vi "Release.vi"(8 "error in (no error)":errorcluster, 11 "Instance":T1) -> (0 "error out":errorcluster, 3 "Children":i32[](array[numeric]))   [LabVIEW 2022 SP3, in "Shared.lvlib"]
uses:
  Shared.lvlib
  Controls/Instance.ctl
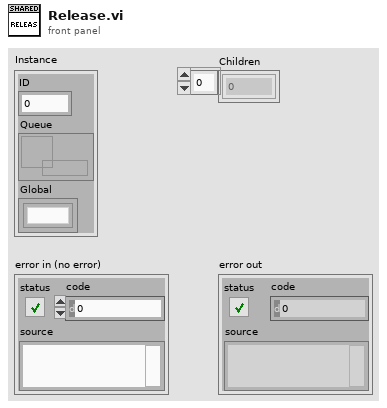
[diagram p1: front panel]
types:
  T1 = typedef "Shared.lvlib/Instance.ctl" = cluster{"ID":i32, "Queue":refnum<queue>, "Global":refnum<k1>}
  T2 = cluster{"ID":i32, "Name":string, "Parent":i32, "Queue":refnum<queue>, "Ini Path":path, "Ini Section":string, "VI Name":string, "VI Path":path, "VI Refnum":refnum<vi>, "Group":string}[]
  T3 = cluster{"ID":i32, "Name":string, "Parent":i32, "Queue":refnum<queue>, "Ini Path":path, "Ini Section":string, "VI Name":string, "VI Path":path, "VI Refnum":refnum<vi>, "Group":string}
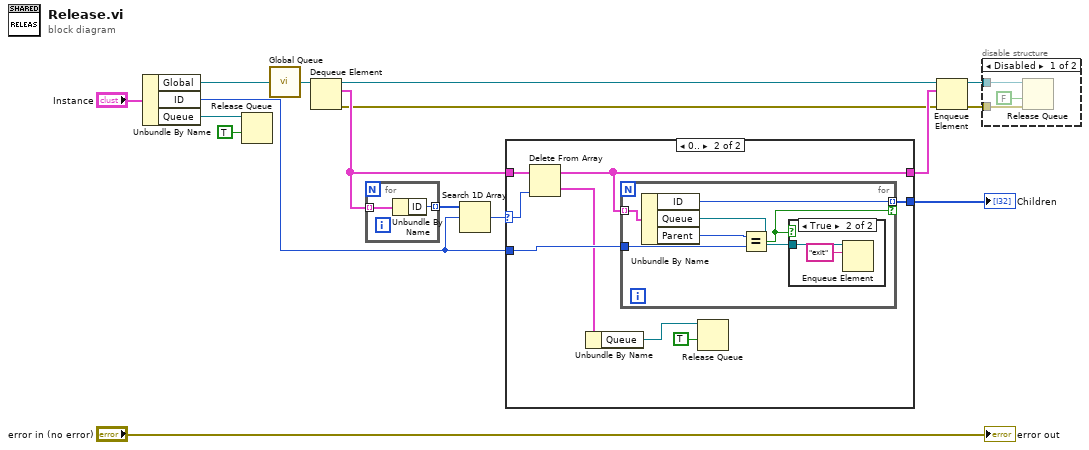
[diagram p0: block diagram]
diagram:
  n1 = Unbundle By Name("Instance") -> ("Global"=w2:refnum<k1>, "ID"=w3:i32, "Queue"=w15:refnum<queue>)
  n2 = Release Queue(queue=w15, force destroy? (F)=TRUE) -> ()  [unwired: 1 in, 3 out]
  n3 = call "Global Queue.vi"("Global in"=w2) -> ("Global"=w1:refnum<queue>)
  n4 = Dequeue Element(queue=w1) -> (queue out=w12:refnum<queue>, element=w10:T2, error out=w5:errorcluster)  [unwired: 2 in, 1 out]
  n5 = for {
    tunnel: w10 -> [w18] mode=indexing
    tunnel: [w17] -> w11 mode=indexing
    n6 = Unbundle By Name(w18) -> ("ID"=w17:i32)
  }
  n7 = Search 1D Array(1D array=w11, element=w3) -> (index of element=w8:i32)  [unwired: 1 in]
  n8 = case shown="0.." w8 {
    selector: w8 -> [_ w26]
    tunnel: w10 -> [w19 w27]
    tunnel: [w19 w25] -> w9
    tunnel: [_ w24] -> w4
    tunnel: w3 -> [_ w23]
    frame ..-1 {
    }
    frame 0.. {
      n9 = Delete From Array(array=w27, index=w26) -> (deleted portion=w22:T3, array with subset deleted=w25:T2)  [unwired: 1 in]
      n10 = Unbundle By Name(w22) -> ("Queue"=w21:refnum<queue>)
      n11 = for {
        tunnel: w25 -> [w33] mode=indexing
        tunnel: [w32] -> w24 mode=indexing if=w28
        tunnel: w23 -> [w30]
        n12 = Unbundle By Name(w33) -> ("ID"=w32:i32, "Queue"=w29:refnum<queue>, "Parent"=w31:i32)
        n13 = Equal?(x=w31, y=w30) -> (x = y?=w28:bool)
        n14 = case shown="True" w28 {
          tunnel: w29 -> [_ w35]
          frame False {
          }
          frame True {
            n15 = Enqueue Element(queue=w35, element="exit") -> ()  [unwired: 2 in, 3 out]
          }
        }
      }
      n16 = Release Queue(queue=w21, force destroy? (F)=TRUE) -> ()  [unwired: 1 in, 3 out]
    }
  }
  "Children" <- w4
  n17 = Enqueue Element(queue=w12, element=w9, error in (no error)=w5) -> (queue out=w7:refnum<queue>, error out=w6:errorcluster)  [unwired: 1 in, 1 out]
  n18 = disable-structure shown="Disabled" {
    disable-tunnel: w7 -> [w38 _]
    disable-tunnel: w6 -> [w37 _]
    frame Disabled {
      n19 = Release Queue(queue=w38, force destroy? (F)=FALSE, error in (no error)=w37) -> ()  [unwired: 3 out]
    }
    frame Enabled {
    }
  }
  "error out" <- "error in (no error)"
